vi "Life_FGV.vi"(7 "Command":enum16{"SET", "GET"}(ring), 8 "error in (no error)":errorcluster, 10 "Error_IN":bool, 11 "Life_Value_IN":dbl) -> (0 "error out":errorcluster, 2 "Error_OUT":bool, 3 "Life_Value_OUT":dbl)   [LabVIEW 2017]
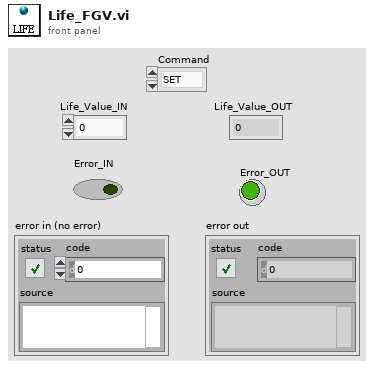
[diagram p1: front panel]
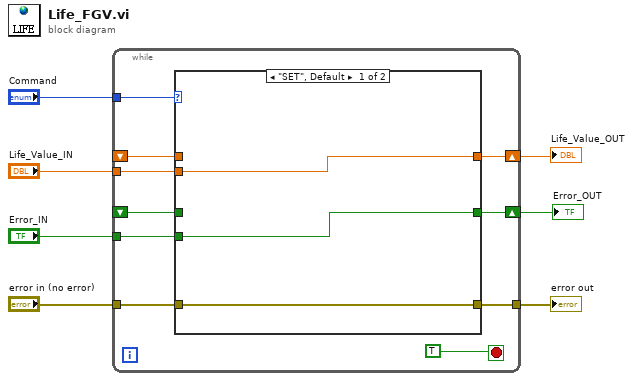
[diagram p0: block diagram]
diagram:
  n1 = while {
    tunnel: "Command" -> [w17]
    shift-right: [w16] -> w6
    shift-left: _ -> [w14]
    tunnel: "Life_Value_IN" -> [w15]
    tunnel: [w12] -> w4
    tunnel: "error in (no error)" -> [w11]
    shift-right: [w10] -> w1
    shift-left: _ -> [w8]
    tunnel: "Error_IN" -> [w9]
    stop <- TRUE stop-if-true
    n2 = case shown="\"SET\", Default" w17 {
      tunnel: [w20 w23] -> w16
      tunnel: w15 -> [w20 _]
      tunnel: w14 -> [_ w23]
      tunnel: [w19 w22] -> w12
      tunnel: w11 -> [w19 w22]
      tunnel: [w18 w21] -> w10
      tunnel: w9 -> [w18 _]
      tunnel: w8 -> [_ w21]
      frame "SET", Default {
      }
      frame "GET" {
      }
    }
  }
  "Life_Value_OUT" <- w6
  "error out" <- w4
  "Error_OUT" <- w1
